vi "Get dates from DB.vi"(10 "Update existing Case":refnum<vi>, 11 "Array":string[](array[string])) -> ()   [LabVIEW 2015]
uses:
  controls/Update Case.ctl
  controls/Program.ctl
  controls/Type.ctl
  controls/Case Status.ctl
  controls/Date.ctl
  controls/Declined.ctl
  controls/Back to Business.ctl
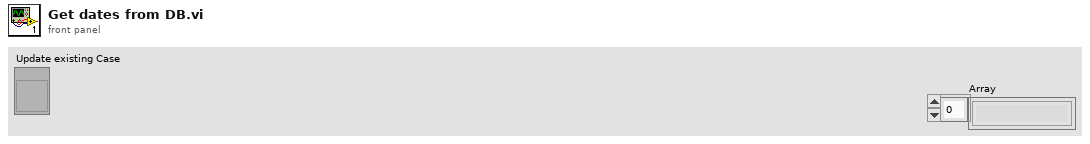
[diagram p1: front panel]
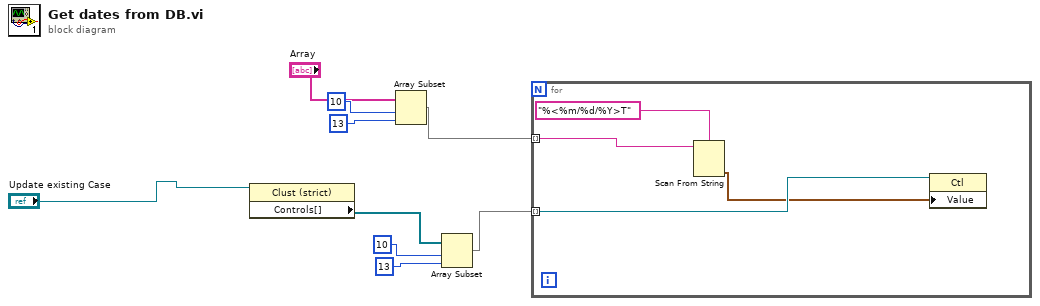
[diagram p0: block diagram]
diagram:
  n1 = property class="Clust (strict)"(reference="Update existing Case") -> ("Controls[]"=w3:refnum<vi>[])  [unwired: 1 in, 2 out]
  n2 = Array Subset(array="Array", index=10, length=13) -> (w6:string[])
  n3 = Array Subset(array=w3, index=10, length=13) -> (w2:refnum<vi>[])
  n4 = for {
    tunnel: w6 -> [w13] mode=indexing
    tunnel: w2 -> [w11] mode=indexing
    n5 = Scan From String(format string="%<%m/%d/%Y>T", input string=w13) -> (output 1=w10:timestamp)  [unwired: 3 in, 3 out]
    n6 = property class="Ctl"(reference=w11, "Value"=w10) -> ()  [unwired: 1 in, 2 out]
  }
